vi "Build Robot IP Address.vi"(1 "Last Byte":u32=2, 2 "In Address":string) -> (0 "Out Address":string)   [LabVIEW 2012, in "femtoRoboLib.lvlib"]
uses:
  femtoRoboLib.lvlib
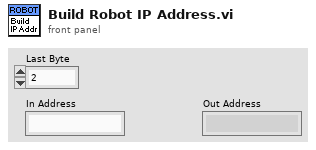
[diagram p1: front panel]
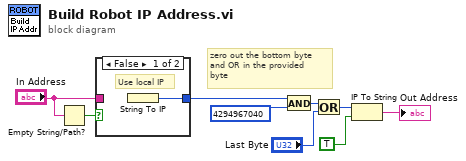
[diagram p0: block diagram]
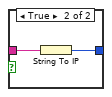
[diagram p2: hidden frame]
diagram:
  # "zero out the bottom byte\nand OR in the provided \nbyte"
  n1 = Empty String/Path?(string/path="In Address") -> (empty?=w7:bool)
  n2 = case shown="False" w7 {
    tunnel: [w10 w12] -> w2
    tunnel: "In Address" -> [_ w11]
    frame False {
      # "Use local IP"
      n3 = String To IP() -> (0:w10:u32)  [unwired: 1 in]
    }
    frame True {
      n4 = String To IP(1:w11) -> (0:w12:u32)
    }
  }
  n5 = And(x=w2, y=u32 4294967040) -> (x .and. y?=w6:u32)
  n6 = Or(x=w6, y="Last Byte") -> (x .or. y?=w3:u32)
  n7 = IP To String(1:TRUE ("dot notation? (F)"), 2:w3) -> (0:→"Out Address":string)
